vi "Configure Device.vi"(8 "error in (no error)":errorcluster, 11 "Simulated Waveform in":refnum<class "Simulated Waveform.lvclass">) -> (0 "error out":errorcluster, 3 "Simulated Waveform out":refnum<class "Simulated Waveform.lvclass">)   [LabVIEW 2020, in "Simulated Waveform.lvlib" / "Simulated Waveform.lvclass"]
uses:
  Simulated Waveform.lvclass
  Simulated Waveform.lvclass/Simulated Waveform.ctl
  build/ppl/Signal Generator.lvlibp/Signal Generator/Signal Generator.lvclass
  build/ppl/lv-hal.lvlibp/Device/Device.lvclass
  C:/dev/HAL Demo/build/ppl/lv-hal.lvlibp/Device/Device.lvclass
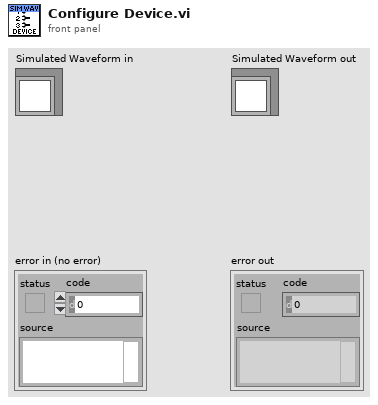
[diagram p1: front panel]
types:
  T1 = typedef "Simulated Waveform.lvlib/Simulated Waveform.lvclass/Ref Data.ctl" = cluster{"Sim Queue Name":string, "Waveform Queue":refnum<queue>, "Noise Factor":dbl}
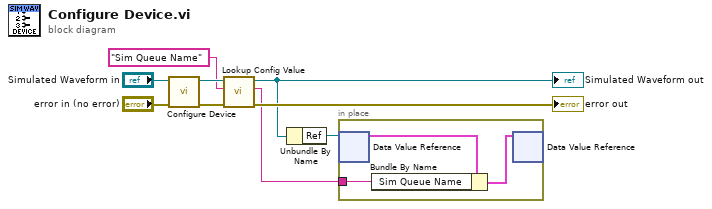
[diagram p0: block diagram]
diagram:
  n1 = call-parent "Configure Device.vi"("error in (no error)"="error in (no error)", "Signal Generator in"="Simulated Waveform in") -> ("error out"=w6:errorcluster, "Signal Generator out"=w7:refnum<class "Simulated Waveform.lvclass">)  [unwired: 8 in]
  n2 = call "Lookup Config Value.vi"("error in (no error)"=w6, "Config Key"="Sim Queue Name", "Device in"=w7) -> ("error out"=→"error out":errorcluster, "Value"=w2:string, "Device out"=w1:refnum<class "Simulated Waveform.lvclass">)  [unwired: 5 in, 1 out]
  "Simulated Waveform out" <- w1
  n3 = Unbundle By Name(w1) -> ("Ref"=w4:refnum<data-value>)
  n4 = in-place {
    in-place-border: w2 -> [w10]
    n5 = in-place-dvr #1(w4) -> (w12:T1)  [unwired: 1 out]
    n6 = Bundle By Name(cluster=w12, "Sim Queue Name"=w10) -> (w11:T1)
    n7 = in-place-dvr #1(w11) -> ()  [unwired: 2 out]
  }
